vi "Stop.vi"(8 "error in (no error)":errorcluster, 11 "1553 Board in":refnum<class "1553 Session.lvclass">) -> (0 "error out":errorcluster, 3 "1553 Board out":refnum<class "1553 Session.lvclass">)   [LabVIEW 2020, in "BCI-1553 API.lvlib" / "1553 Session.lvclass"]
doc: "Stops a 1553 Session if it is already started."
uses:
  1553 Session.lvclass
  1553 Session.lvclass/1553 Session.ctl
  1553 Component/1553 Component.lvclass
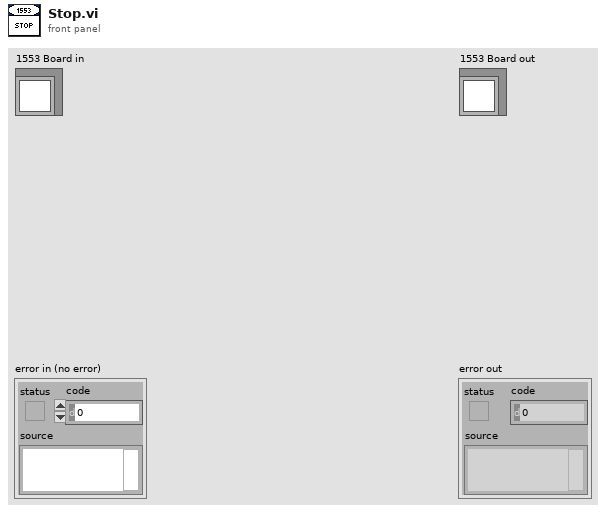
[diagram p1: front panel]
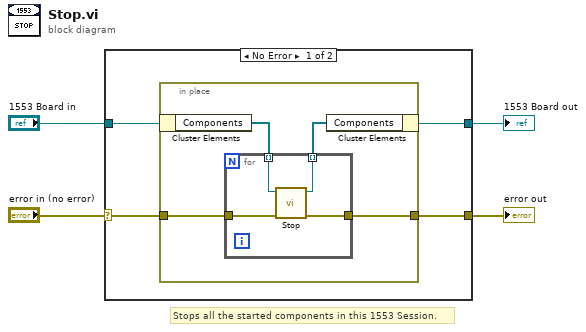
[diagram p0: block diagram]
diagram:
  # "Stops all the started components in this 1553 Session."
  n1 = case shown="No Error" "error in (no error)" {
    selector: "error in (no error)" -> [w7 w18]
    tunnel: [w6 w18] -> w2
    tunnel: [w5 w17] -> w1
    tunnel: "1553 Board in" -> [w8 w17]
    frame No Error {
      n2 = in-place {
        in-place-border: w7 -> [w12]
        in-place-border: [w9] -> w6
        n3 = in-place-cluster #1(w8) -> ("Components"=w11:refnum<class "1553 Component.lvclass">[])
        n4 = for {
          tunnel: w12 -> [w15]
          tunnel: [w14] -> w9
          tunnel: w11 -> [w16] mode=indexing
          tunnel: [w13] -> w10 mode=indexing
          n5 = call-dynamic "Stop.vi"("error in (no error)"=w15, "1553 Component in"=w16) -> ("error out"=w14:errorcluster, "1553 Component out"=w13:refnum<class "1553 Component.lvclass">)  [unwired: 8 in]
        }
        n6 = in-place-cluster #1("Components"=w10) -> (w5:refnum<class "1553 Session.lvclass">)
      }
    }
    frame Error {
    }
  }
  "error out" <- w2
  "1553 Board out" <- w1
